vi "get index type definitions.vi"(11 "Temperature Controller Logic configuration in":refnum<class "Temperature Controller Logic configuration.lvclass">) -> (2 "index type defs":T1, 3 "Temperature Controller Logic configuration out":refnum<class "Temperature Controller Logic configuration.lvclass">)   [LabVIEW 2013, in "Temperature Controller Logic configuration.lvclass"]
uses:
  Temperature Controller Logic configuration.lvclass
  <vilib>/NI/Tag Bus Data Framework/fixed module parent/module/configuration/index type definitions.ctl
  input data indices.ctl
  output data indices.ctl
  parameter data indices.ctl
  result data indices.ctl
  <vilib>/NI/Tag Bus Data Framework/fixed module parent/module/configuration/fixed channel configuration.lvclass
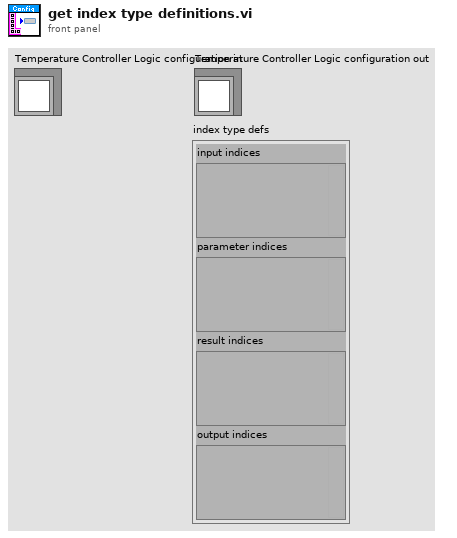
[diagram p1: front panel]
types:
  T1 = typedef "fixed channel configuration.lvclass/index type definitions.ctl" = cluster{"input indices":variant, "parameter indices":variant, "result indices":variant, "output indices":variant}
  T2 = typedef "Temperature Controller Logic configuration.lvclass/result data indices.ctl" = cluster{"Double.fan":i32, "Double.lamp":i32}
  T3 = typedef "Temperature Controller Logic configuration.lvclass/parameter data indices.ctl" = cluster{"Double.Temperature":i32, "Double.setpoint":i32, "Double.output range high":i32, "Double.output range low":i32, "Double.Kc":i32, "Double.Ti":i32, "Double.Td":i32, "Boolean.Fan on?":i32}
  T4 = typedef "Temperature Controller Logic configuration.lvclass/output data indices.ctl" = cluster{"placeholder":i32}
  T5 = typedef "Temperature Controller Logic configuration.lvclass/input data indices.ctl" = cluster{"placeholder":i32}
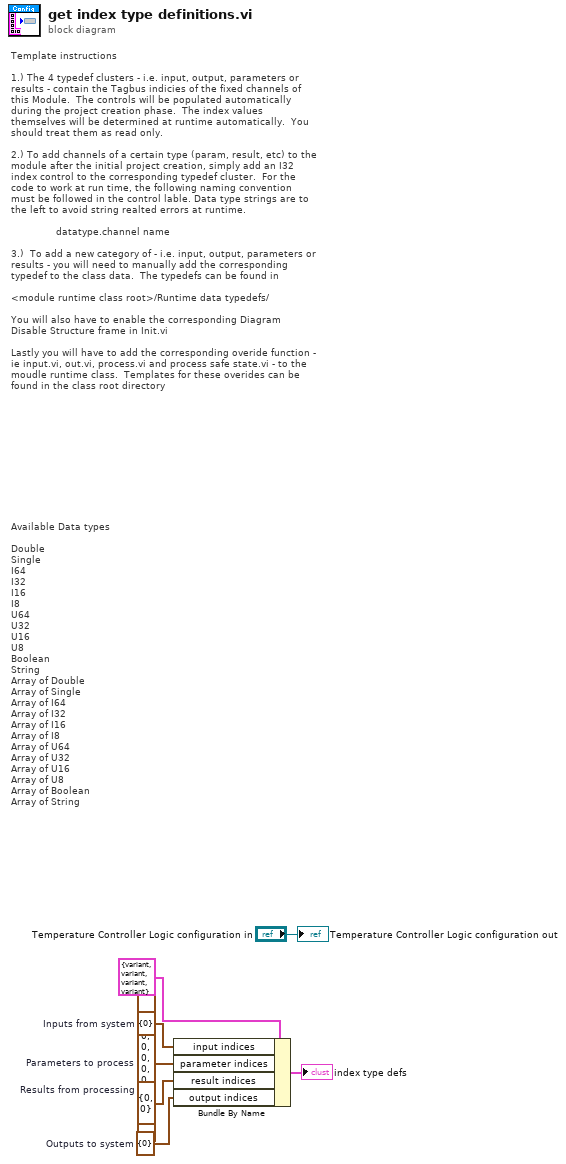
[diagram p0: block diagram]
diagram:
  w4 = T2 {"Double.fan"=0, "Double.lamp"=0}  # Results from processing
  w3 = T3 {"Double.Temperature"=0, "Double.setpoint"=0, "Double.output range high"=0, "Double.output range low"=0, "Double.Kc"=0, "Double.Ti"=0, "Double.Td"=0, "Boolean.Fan on?"=0}  # Parameters to process
  w2 = T4 {"placeholder"=0}  # Outputs to system
  w1 = T5 {"placeholder"=0}  # Inputs from system
  # "Available Data types\n\nDouble\nSingle\nI64\nI32\nI16\nI8\nU64\nU32\nU16\nU8\nBoolean\nString\nArray of Double\nArray of Single\nArray of I64\nArray of I32\nArray of I16\nArray of I8\nArray of U64\nArray of U32\nArray of U16\nArray of U8\nArray of Boolean\nArray of String"
  # "Template instructions\n\n1.) The 4 typedef clusters - i.e. input, output, parameters or results - contain the Tagbus indicies of the fixed channels of this Module.  The controls will be populated automatically during the project creation phase.  The index values themselves will be determined at runtime automatically.  You should treat them as read only.\n\n2.) To add channels of a certain type (param, result, etc) to the module after the initial project creation, simply add an I32 index control to the corresponding typedef cluster.  For the code to work at run time, the following naming convention must be followed in the control lable. Data type strings are to the left to avoid string realted errors at runtime.\n\n               datatype.channel name\n\n3.)  To add a new category of - i.e. input, output, parameters or results - you will need to manually add the corresponding typedef to the class data.  The typedefs can be found in \n\n<module runtime class root>/Runtime data typedefs/\n\nYou will also have to enable the corresponding Diagram Disable Structure frame in Init.vi\n\nLastly you will have to add the corresponding overide function - ie input.vi, out.vi, process.vi and process safe state.vi - to the moudle runtime class.  Templates for these overides can be found in the class root directory"
  n1 = Bundle By Name(cluster=T1 {"input indices"=variant, "parameter indices"=variant, "result indices"=variant, "output indices"=variant} ("index type defs"), "input indices"=w1, "parameter indices"=w3, "result indices"=w4, "output indices"=w2) -> (→"index type defs":T1)
  "Temperature Controller Logic configuration out" <- "Temperature Controller Logic configuration in"
